vi "DoInit.vi"(8 "error in (no error)":errorcluster, 11 "Menu in":refnum<class "Menu.lvclass">) -> (0 "error out":errorcluster, 3 "Menu out":refnum<class "Menu.lvclass">)   [LabVIEW 2019, in "RT_Game.lvlib" / "Menu.lvclass"]
uses:
  Menu.lvclass
  C:/Users/FreshBob/Dropbox/VIs/myRIO_GameConsole/RT/RT_Game/Game/Game.lvclass
  Game/Coordinate.ctl
  Menu.lvclass/Menu.ctl
  Game/Game.lvclass
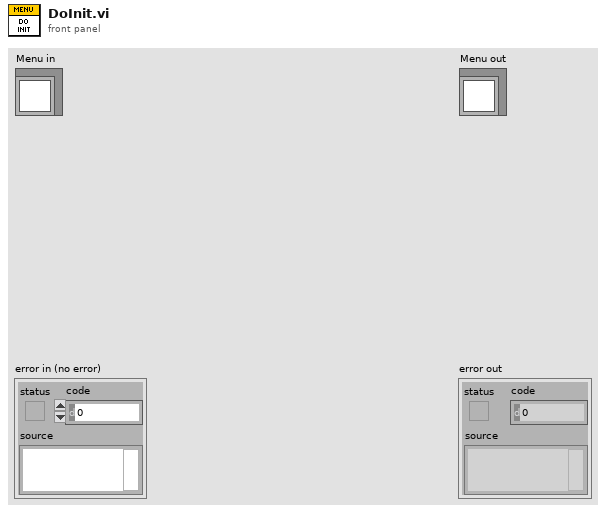
[diagram p1: front panel]
types:
  T1 = typedef "RT_Game.lvlib/Game.lvclass/Coordinate.ctl" = cluster{"x":dbl, "y":dbl}
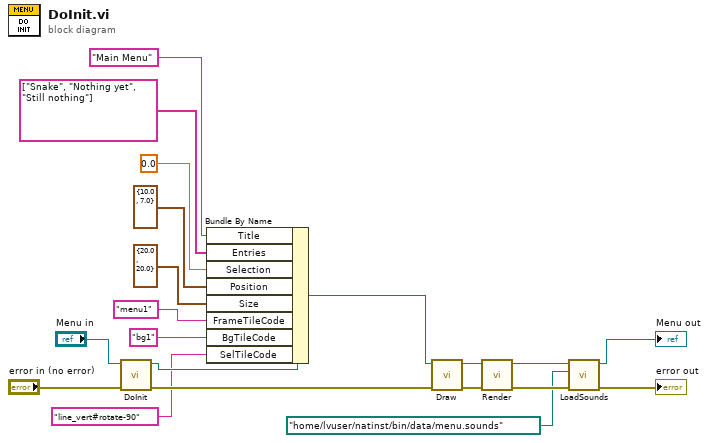
[diagram p0: block diagram]
diagram:
  n1 = call-parent "DoInit.vi"("error in (no error)"="error in (no error)", "Game in"="Menu in") -> ("error out"=w20:errorcluster, "Game out"=w17:refnum<class "Menu.lvclass">)  [unwired: 8 in]
  n2 = Bundle By Name(cluster=w17, "Title"="Main Menu", "Entries"=string[] ["Snake", "Nothing yet", "Still nothing"], "Selection"=0.0, "Position"=T1 {"x"=10.0, "y"=7.0}, "Size"=T1 {"x"=20.0, "y"=20.0}, "FrameTileCode"="menu1", "BgTileCode"="bg1", "SelTileCode"="line_vert#rotate-90") -> (w7:refnum<class "Menu.lvclass">)
  n3 = call "Draw.vi"("error in (no error)"=w20, "Menu in"=w7) -> ("error out"=w8:errorcluster, "Menu out"=w5:refnum<class "Menu.lvclass">)  [unwired: 8 in]
  n4 = call-dynamic "Render.vi"("error in (no error)"=w8, "Game in"=w5) -> ("error out"=w6:errorcluster, "Game out"=w3:refnum<class "Menu.lvclass">)  [unwired: 8 in]
  n5 = call "LoadSounds.vi"("error in (no error)"=w6, "Path"=path "/home/lvuser/natinst/bin/data/menu.sounds", "Game in"=w3) -> ("error out"=→"error out":errorcluster, "Game out"=→"Menu out":refnum<class "Menu.lvclass">)  [unwired: 7 in]
